vi "Read All Properties.vi"(6 "timeout (ms)":i32=-1, 8 "error in (no error)":errorcluster, 11 "FlexLogger_gRPCAPI in":refnum<class "FlexLogger_gRPC.lvclass">) -> (0 "error out":errorcluster, 2 "Test_Properties Array":T1[](array[typedef]), 3 "FlexLogger_gRPCAPI out":refnum<class "FlexLogger_gRPC.lvclass">)   [LabVIEW 2020, in "FlexLogger_gRPC.lvlib" / "FlexLogger_gRPC.lvclass"]
uses:
  FlexLogger_gRPC.lvclass
  Controls/test_property Type.ctl
  FlexLogger_client/RPC Messages/flexlogger_GetTestPropertiesRequest.ctl
  FlexLogger_client/RPC Messages/flexlogger_ElementIdentifier.ctl
  FlexLogger_gRPC.lvclass/FlexLogger_gRPC.ctl
  FlexLogger_client/FlexLogger_client.lvlib
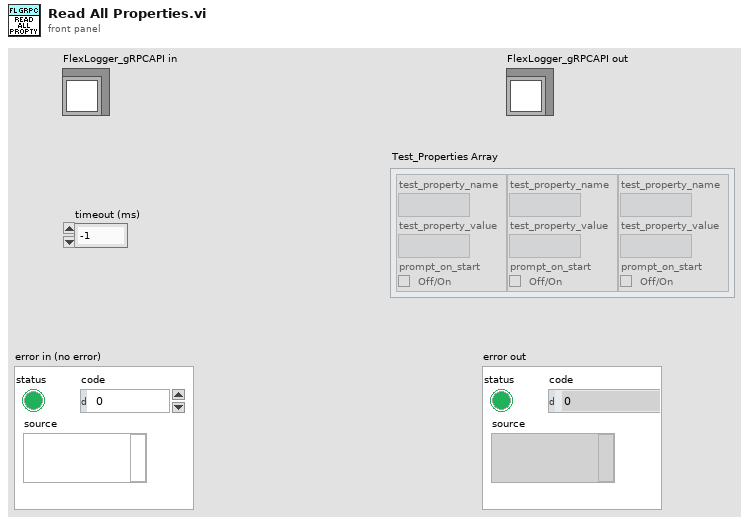
[diagram p1: front panel]
types:
  T1 = typedef "FlexLogger_gRPC.lvlib/FlexLogger_gRPC.lvclass/test_property Type.ctl" = cluster{"test_property_name":string, "test_property_value":string, "prompt_on_start":bool}
  T2 = typedef "FlexLogger_client.lvlib/flexlogger_GetTestPropertiesRequest.ctl" = cluster{"document_identifier":T3}
  T3 = typedef "FlexLogger_client.lvlib/flexlogger_ElementIdentifier.ctl" = cluster{"project_id":string, "file_name":string, "element_id":string, "subpart_id":string}
  T4 = typedef "grpc-lvsupport-release.lvlib/grpcId.ctl" = u64
  T5 = typedef "FlexLogger_client.lvlib/flexlogger_GetTestPropertiesResponse.ctl" = cluster{"test_properties":T6[]}
  T6 = typedef "FlexLogger_client.lvlib/flexlogger_TestProperty.ctl" = cluster{"property_name":string, "property_value":string, "prompt_on_start":bool}
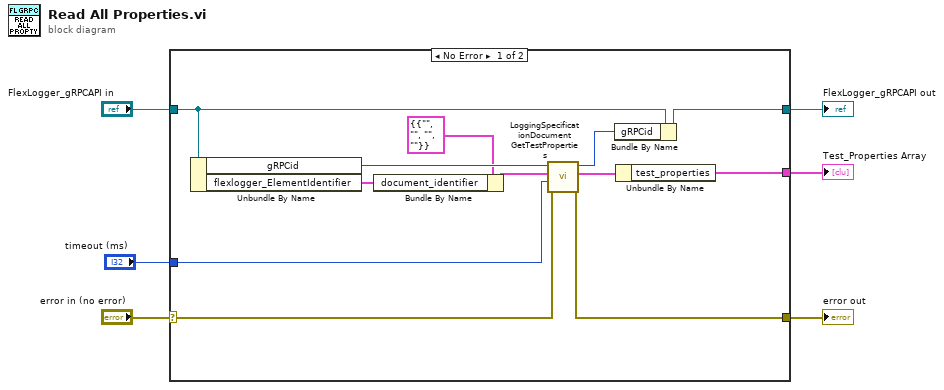
[diagram p0: block diagram]
diagram:
  n1 = case shown="No Error" "error in (no error)" {
    selector: "error in (no error)" -> [w11 w19]
    tunnel: [w17 _] -> w5
    tunnel: "FlexLogger_gRPCAPI in" -> [w15 w20]
    tunnel: [w14 w20] -> w3
    tunnel: [w13 w19] -> w2
    tunnel: "timeout (ms)" -> [w7 _]
    frame No Error {
      n2 = Unbundle By Name(w15) -> ("gRPCid"=w12:T4, "flexlogger_ElementIdentifier"=w8:T3)
      n3 = Bundle By Name(cluster=T2 {"document_identifier"={"project_id"="", "file_name"="", "element_id"="", "subpart_id"=""}} ("Request Data"), "document_identifier"=w8) -> (w9:T2)
      n4 = call "LoggingSpecificationDocument GetTestProperties.vi"("error in"=w11, "timeout (ms)"=w7, "Request Data"=w9, "gRPC ID"=w12) -> ("error out"=w13:errorcluster, "Response Data"=w18:T5, "gRPC ID out"=w16:T4)  [unwired: 5 in]
      n5 = Bundle By Name(cluster=w15, "gRPCid"=w16) -> (w14:refnum<class "FlexLogger_gRPC.lvclass">)
      n6 = Unbundle By Name(w18) -> ("test_properties"=w17:T6[])
    }
    frame Error {
    }
  }
  "error out" <- w2
  "FlexLogger_gRPCAPI out" <- w3
  "Test_Properties Array" <- w5
